vi "parse CSV file for tags.vi"() -> (1 "create tags?":bool, 2 "create channels?":bool, 3 "tags":T1[](array[typedef]), 5 "outputs?":bool[](array[boolean]))   [LabVIEW 2013, in "EIP Tags editor node.lvclass"]
uses:
  EIP Tags editor node.lvclass
  configuration/eip tag definition.ctl
  configuration/eip tag types.ctl
  configuration/EIP Tags Configuration.lvclass
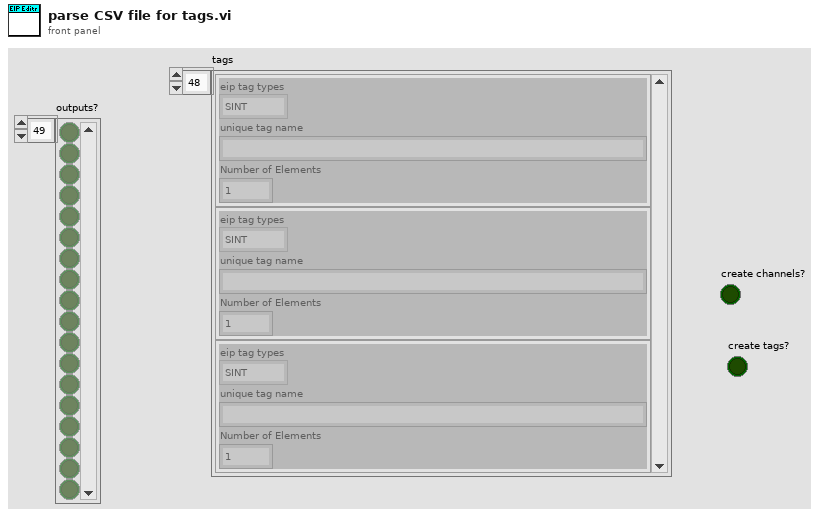
[diagram p1: front panel]
types:
  T1 = typedef "EIP Tags Configuration.lvclass/eip tag definition.ctl" = cluster{"eip tag types":T2, "unique tag name":string, "Number of Elements":u32}
  T2 = typedef "EIP Tags Configuration.lvclass/eip tag types.ctl" = enum16{"SINT", "INT", "DINT", "REAL", "BOOL", "STRING"}
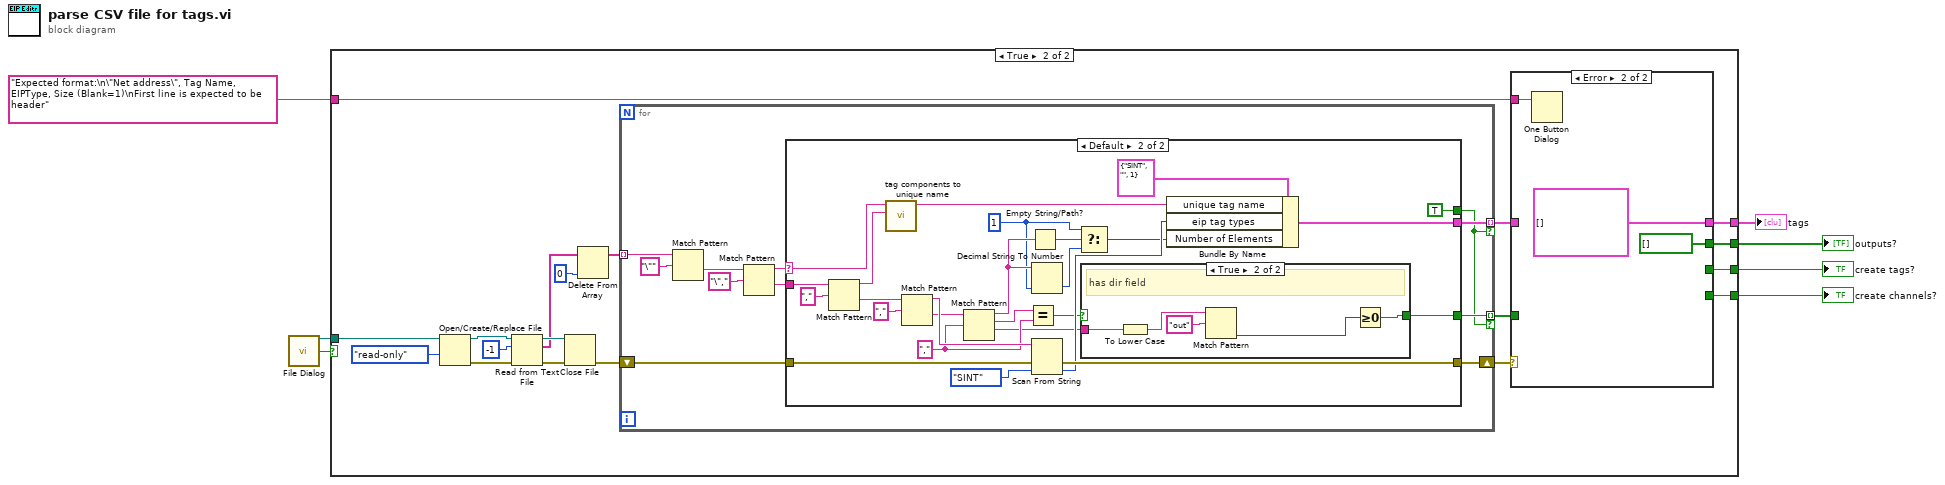
[diagram p0: block diagram]
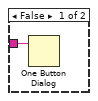
[diagram p2: hidden frame]
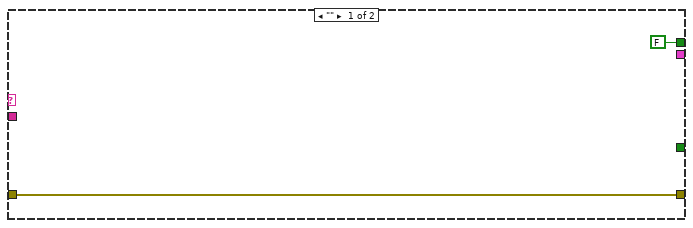
[diagram p3: hidden frame]
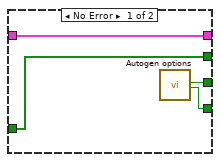
[diagram p5: hidden frame]
diagram:
  n1 = call "File Dialog"() -> ("selected path"=w3:path, "exists"=w4:bool)  [unwired: 12 in, 2 out]
  n2 = case shown="True" w4 {
    tunnel: [_ w27] -> w7
    tunnel: [_ w26] -> w6
    tunnel: [_ w25] -> w5
    tunnel: w3 -> [_ w22]
    tunnel: "Expected format:\n\"Net address\", Tag Name, EIPType, Size (Blank=1)\nFirst line is expected to be header" ("message") -> [w8 w24]
    tunnel: [_ w9] -> w1
    frame False {
      n3 = One Button Dialog(message=w8) -> ()  [unwired: 1 in, 1 out]
    }
    frame True {
      n4 = Open/Create/Replace File(file path (use dialog)=w22, access (0:read/write)=enum16{"read/write", "read-only", "write-only"}."read-only") -> (refnum out=w20:refnum<file>, error out=w21:errorcluster)  [unwired: 4 in, 1 out]
      n5 = Read from Text File(file (use dialog)=w20, count=-1, error in=w21) -> (refnum out=w18:refnum<file>, text=w14:string[], error out=w17:errorcluster)  [unwired: 1 in, 1 out]
      n6 = Close File(refnum=w18, error in=w17) -> (error out=w16:errorcluster)  [unwired: 1 out]
      n7 = Delete From Array(array=w14, index=0) -> (array with subset deleted=w13:string[])  [unwired: 1 in, 1 out]
      n8 = for {
        shift-right: [w31] -> w12
        shift-left: w16 -> [w32]
        tunnel: w13 -> [w37] mode=indexing
        tunnel: [w38] -> w11 mode=indexing if=w28
        tunnel: [w29] -> w10 mode=indexing if=w28
        n9 = Match Pattern(string=w37, regular expression="\"") -> (after substring=w35:string)  [unwired: 1 in, 3 out]
        n10 = Match Pattern(string=w35, regular expression="\",") -> (before substring=w30:string, after substring=w33:string)  [unwired: 1 in, 2 out]
        n11 = case shown="Default" w30 {
          selector: w30 -> [_ w53]
          tunnel: [_ w65] -> w38
          tunnel: w33 -> [_ w63]
          tunnel: w32 -> [w39 w58]
          tunnel: [w39 w57] -> w31
          tunnel: [FALSE TRUE] -> w28
          tunnel: [_ w41] -> w29
          frame "" {
          }
          frame Default {
            w49 = "," ("regular expression")
            w44 = u32 1 ("Number of Elements")
            n12 = Match Pattern(string=w63, regular expression=",") -> (before substring=w59:string, after substring=w61:string)  [unwired: 1 in, 2 out]
            n13 = call "tag components to unique name.vi"("Tag Name"=w59, "Network Path"=w53) -> ("unique name"=w64:string)  [unwired: 9 in]
            n14 = Match Pattern(string=w61, regular expression=",") -> (before substring=w56:string, after substring=w51:string)  [unwired: 1 in, 2 out]
            n15 = Match Pattern(string=w51, regular expression=w49) -> (before substring=w45:string, match substring=w50:string, after substring=w47:string)  [unwired: 1 in, 1 out]
            n16 = Equal?(x=w50, y=w49) -> (x = y?=w48:bool)
            n17 = Empty String/Path?(string/path=w45) -> (empty?=w46:bool)
            n18 = Decimal String To Number(string=w45, default (0L)=w44) -> (number=w43:u32)  [unwired: 1 in, 1 out]
            n19 = Scan From String(input string=w56, error in=w58, default 1=eip_tag_types."SINT" ("eip tag types")) -> (error out=w57:errorcluster, output 1=w54:T2)  [unwired: 2 in, 2 out]
            n20 = Select(t=w44, s=w46, f=w43) -> (s? t:f=w42:u32)
            n21 = case shown="True" w48 {
              selector: w48 -> [w67 _]
              tunnel: w47 -> [_ w72]
              tunnel: [w67 w68] -> w41
              frame False {
                # "f=input, a safe default"
                # "no dir"
              }
              frame True {
                # "has dir field"
                n22 = To Lower Case(string=w72) -> (all lower case string=w71:string)
                n23 = Match Pattern(string=w71, regular expression="out") -> (offset past match=w69:i32)  [unwired: 1 in, 3 out]
                n24 = Greater Or Equal To 0?(x=w69) -> (x >= 0?=w68:bool)
              }
            }
            n25 = Bundle By Name(cluster=T1 {"eip tag types"=enum."SINT", "unique tag name"="", "Number of Elements"=1} ("tag spec"), "unique tag name"=w64, "eip tag types"=w54, "Number of Elements"=w42) -> (w65:T1)
          }
        }
      }
      n26 = case shown="Error" w12 {
        tunnel: [w76 _] -> w27
        tunnel: [w75 _] -> w26
        tunnel: [w74 T1[] [] ("tags 2")] -> w25
        tunnel: w24 -> [_ w78]
        tunnel: w11 -> [w74 _]
        tunnel: w10 -> [w73 _]
        tunnel: [w73 bool[] []] -> w9
        frame No Error {
          n27 = call "Autogen options"() -> ("Map Channels to Tags"=w75:bool, "Create Channels"=w76:bool)  [unwired: 16 in, 2 out]
        }
        frame Error {
          n28 = One Button Dialog(message=w78) -> ()  [unwired: 1 in, 1 out]
        }
      }
    }
  }
  "tags" <- w5
  "create channels?" <- w7
  "create tags?" <- w6
  "outputs?" <- w1
